vi "读取B版外设配置.vi"(8 "error in (no error)":errorcluster, 11 "MB session in":refnum<class "MB_Master.lvclass">) -> (0 "error out":errorcluster, 2 "外设配置":T1 {"阀型号" items=["垦拓10通阀"]; "总氮x公式0" items=["0", "1"]; "光谱仪类型" items=["1型", "2型", "3型", "2型氙灯联控"]; "泵类型" items=["润泽注射泵", "垦拓注射泵"]}, 3 "MB session out":refnum<class "MB_Master.lvclass">)   [LabVIEW 2016, in "斯坦道氨氮.lvlib"]
uses:
  <vilib>/Plasmionique/MB Master/MB_Master/MB_Master.lvclass
  <vilib>/Plasmionique/MB Master/MB_Master_Serial/MB_Master_Serial.lvclass
  D:/Program Files (x86)/National Instruments/LabVIEW 2016/vi.lib/Plasmionique/MB Master/MB_Master/MB_Master.lvclass
  <vilib>/Plasmionique/MB Master/MB Master.lvlib
panel:
  in  "VISA Resource":refnum<visa-resource-name>
  in  "引用选择":enum16{"MB引用", "自建引用"}(ring)
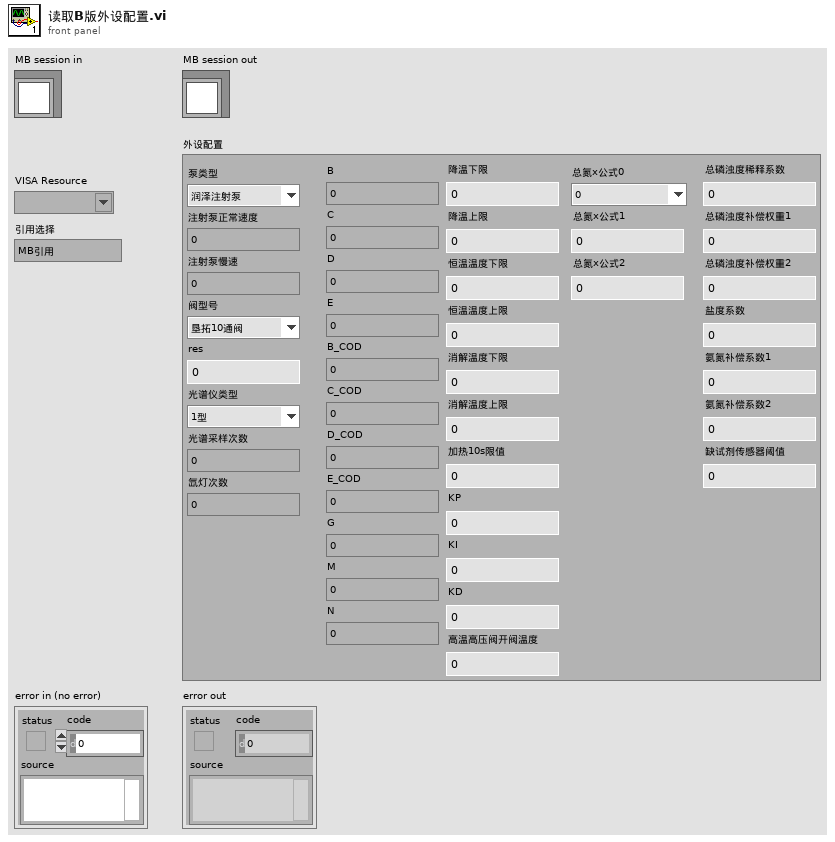
[diagram p1: front panel]
types:
  T1 = typedef "斯坦道氨氮.lvlib/V3 B版外设参数.ctl" = cluster{"泵类型":u8, "注射泵正常速度":u32, "注射泵慢速":u32, "阀型号":u8, "res":u8, "光谱仪类型":u8, "光谱采样次数":u8, "氙灯次数":u8, "B":u16, "C":u16, "D":u16, "E":u16, "B_COD":u16, "C_COD":u16, "D_COD":u16, "E_COD":u16, "G":u16, "M":u16, "N":u16, "降温下限":sgl, "降温上限":sgl, "恒温温度下限":sgl, "恒温温度上限":sgl, "消解温度下限":sgl, "消解温度上限":sgl, "加热10s限值":sgl, "KP":sgl, "KI":sgl, "KD":sgl, "高温高压阀开阀温度":sgl, "总氮x公式0":u8, "总氮x公式1":sgl, "总氮x公式2":sgl, "总磷浊度稀释系数":sgl, "总磷浊度补偿权重1":sgl, "总磷浊度补偿权重2":sgl, "盐度系数":sgl, "氨氮补偿系数1":sgl, "氨氮补偿系数2":sgl, "缺试剂传感器阈值":u16}
  T2 = cluster{"baud rate (bps)":u32, "stop bits":u16, "parity":u16, "flow control":u16, "timeout":u32, "retries":i32}
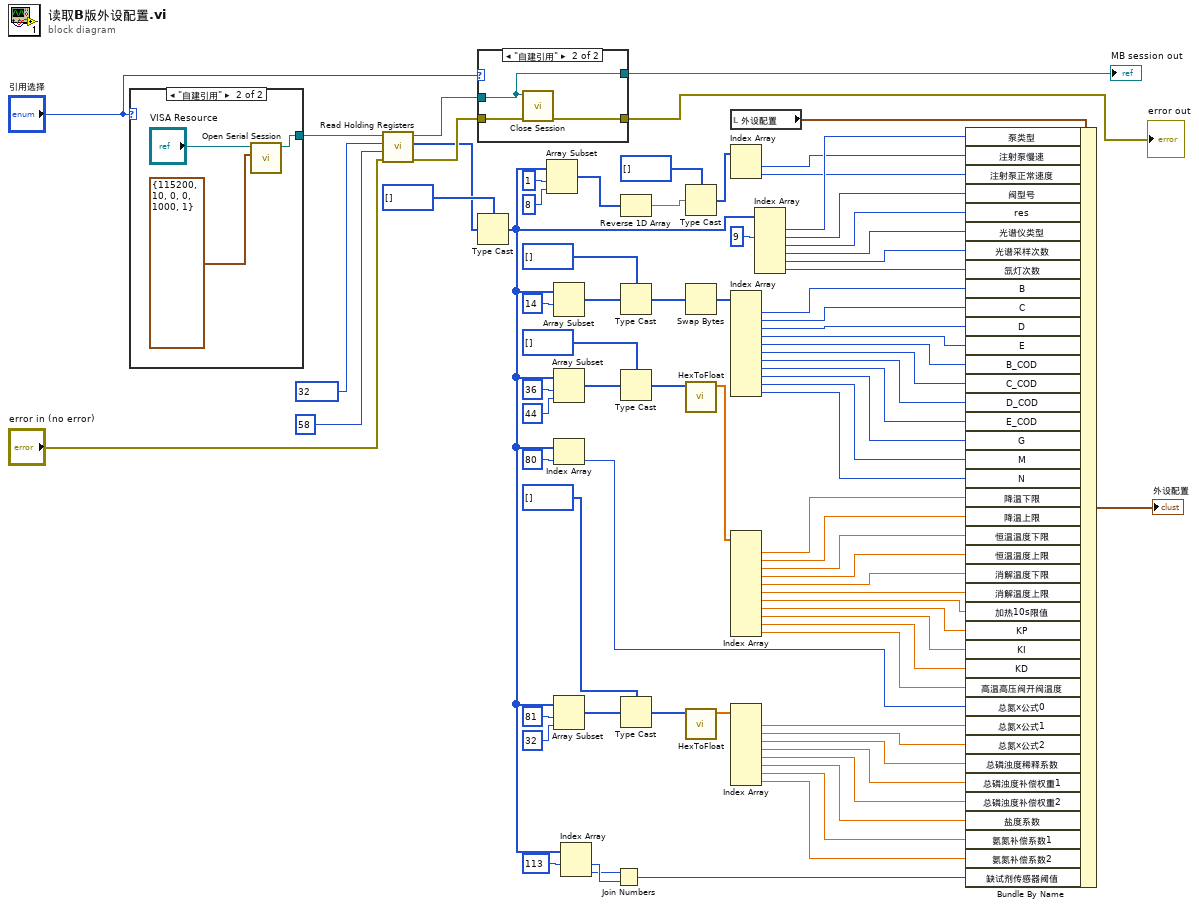
[diagram p0: block diagram]
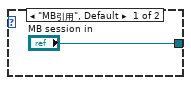
[diagram p3: hidden frame]
diagram:
  n1 = case shown="\"自建引用\"" "引用选择" {
    tunnel: ["MB session in" w86] -> w72
    frame "MB引用", Default {
    }
    frame "自建引用" {
      n2 = call <vilib>:"Open Serial Session.vi"("Serial Config"=T2 {"baud rate (bps)"=115200, "stop bits"=10, "parity"=0, "flow control"=0, "timeout"=1000, "retries"=1}, "VISA Resource"="VISA Resource") -> ("MB_Serial session"=w86:refnum<class "MB_Master_Serial.lvclass">)  [unwired: 8 in, 1 out]
    }
  }
  n3 = call <vilib>:"Read Holding Registers.vi"("error in (no error)"="error in (no error)", "quantity"=u16 58, "starting address"=u16 32, "MB session in"=w72) -> ("error out"=w69:errorcluster, "Registers"=w48:u16[], "MB session out"=w71:refnum<class "MB_Master.lvclass">)  [unwired: 5 in]
  n4 = case shown="\"自建引用\"" "引用选择" {
    tunnel: w71 -> [w87 w89]
    tunnel: w69 -> [w88 w91]
    tunnel: [w88 w90] -> w68
    tunnel: [w87 w89] -> w67
    frame "MB引用", Default {
    }
    frame "自建引用" {
      n5 = call-dynamic "Close Session.vi"("error in (no error)"=w91, "MB session in"=w89) -> ("error out"=w90:errorcluster)  [unwired: 9 in]
    }
  }
  "MB session out" <- w67
  "error out" <- w68
  n6 = Type Cast(type=u8[] [], x=w48) -> (*(type *) &x=w5:u8[])
  n7 = Array Subset(array=w5, index=1 ("索引"), length=8 ("长度")) -> (w76:u8[])
  n8 = Array Subset(array=w5, index=14 ("索引")) -> (w58:u8[])  [unwired: 1 in]
  n9 = Array Subset(array=w5, index=36 ("索引"), length=44 ("长度")) -> (w63:u8[])
  n10 = Index Array(array=w5, index=80 ("索引")) -> (element=w15:u8)
  n11 = Array Subset(array=w5, index=81 ("索引"), length=32 ("长度")) -> (w53:u8[])
  n12 = Index Array(array=w5, index #1=113 ("索引")) -> (element #1=w3:u8, element #2=w2:u8)  [unwired: 1 in]
  n13 = Join Numbers(hi=w2, lo=w3) -> ((hi.lo)=w1:u16)
  n14 = Reverse 1D Array(array=w76) -> (reversed array=w75:u8[])
  n15 = Type Cast(type=u16[] [], x=w58) -> (*(type *) &x=w57:u16[])
  n16 = Type Cast(type=u16[] [], x=w63) -> (*(type *) &x=w61:u16[])
  n17 = Type Cast(type=u16[] [], x=w53) -> (*(type *) &x=w52:u16[])
  n18 = Type Cast(type=u32[] [], x=w75) -> (*(type *) &x=w73:u32[])
  n19 = Swap Bytes(anything=w57) -> (byte swapped=w56:u16[])
  n20 = call "HexToFloat.vi"("数组"=w61) -> ("FLOAT"=w64:sgl[])  [unwired: 10 in]
  n21 = call "HexToFloat.vi"("数组"=w52) -> ("FLOAT"=w54:sgl[])  [unwired: 10 in]
  n22 = local read "外设配置"() -> (w47:T1)
  n23 = Index Array(array=w73) -> (element #1=w44:u32, element #2=w43:u32)  [unwired: 2 in]
  n24 = Index Array(array=w56) -> (element #1=w37:u16, element #2=w36:u16, element #3=w35:u16, element #4=w34:u16, element #5=w33:u16, element #6=w32:u16, element #7=w31:u16, element #8=w30:u16, element #9=w29:u16, element #10=w28:u16, element #11=w27:u16)  [unwired: 11 in]
  n25 = Index Array(array=w64) -> (element #1=w26:sgl, element #2=w25:sgl, element #3=w24:sgl, element #4=w23:sgl, element #5=w22:sgl, element #6=w21:sgl, element #7=w20:sgl, element #8=w19:sgl, element #9=w18:sgl, element #10=w17:sgl, element #11=w16:sgl)  [unwired: 11 in]
  n26 = Index Array(array=w54) -> (element #1=w14:sgl, element #2=w13:sgl, element #3=w12:sgl, element #4=w11:sgl, element #5=w10:sgl, element #6=w9:sgl, element #7=w8:sgl, element #8=w7:sgl)  [unwired: 8 in]
  n27 = Index Array(array=w5, index #2=9 ("索引")) -> (element #1=w45:u8, element #2=w42:u8, element #3=w41:u8, element #4=w40:u8, element #5=w39:u8, element #6=w38:u8)  [unwired: 5 in]
  n28 = Bundle By Name(cluster=w47, "泵类型"=w45, "注射泵慢速"=w44, "注射泵正常速度"=w43, "阀型号"=w42, "res"=w41, "光谱仪类型"=w40, "光谱采样次数"=w39, "氙灯次数"=w38, "B"=w37, "C"=w36, "D"=w35, "E"=w34, "B_COD"=w33, "C_COD"=w32, "D_COD"=w31, "E_COD"=w30, "G"=w29, "M"=w28, "N"=w27, "降温下限"=w26, "降温上限"=w25, "恒温温度下限"=w24, "恒温温度上限"=w23, "消解温度下限"=w22, "消解温度上限"=w21, "加热10s限值"=w20, "KP"=w19, "KI"=w18, "KD"=w17, "高温高压阀开阀温度"=w16, "总氮x公式0"=w15, "总氮x公式1"=w14, "总氮x公式2"=w13, "总磷浊度稀释系数"=w12, "总磷浊度补偿权重1"=w11, "总磷浊度补偿权重2"=w10, "盐度系数"=w9, "氨氮补偿系数1"=w8, "氨氮补偿系数2"=w7, "缺试剂传感器阈值"=w1) -> (→"外设配置":T1)
